vi "POST.vi"(6 "timeout":i32=10000, 7 "output file":path, 8 "error in":errorcluster, 9 "buffer":string, 10 "url":string, 11 "http-client in":refnum<class "http-client.lvclass">) -> (0 "error out":errorcluster, 1 "body":string, 2 "headers":string, 3 "http-client out":refnum<class "http-client.lvclass">)   [LabVIEW 2020, in "REST Client.lvlib" / "http-client.lvclass"]
uses:
  http-client.lvclass
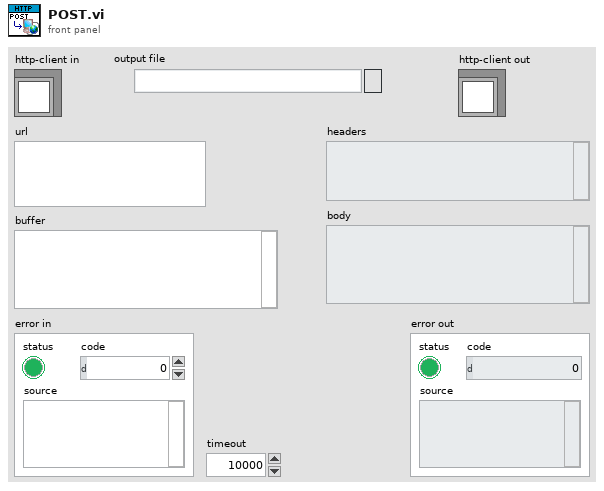
[diagram p1: front panel]
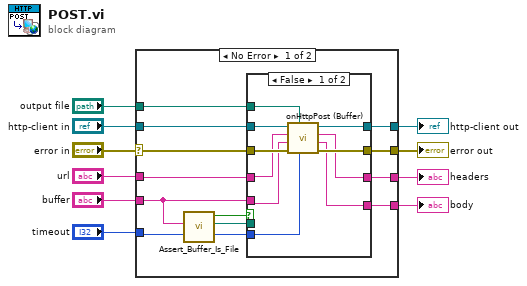
[diagram p0: block diagram]
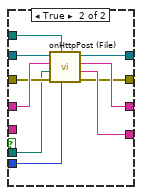
[diagram p2: hidden frame]
diagram:
  n1 = case shown="No Error" "error in" {
    selector: "error in" -> [w11 w44]
    tunnel: [w12 w44] -> w9
    tunnel: [w17 w43] -> w7
    tunnel: "http-client in" -> [w19 w43]
    tunnel: [w16 _] -> w6
    tunnel: "url" -> [w13 _]
    tunnel: "timeout" -> [w14 _]
    tunnel: "output file" -> [w18 _]
    tunnel: [w15 _] -> w2
    tunnel: "buffer" -> [w20 _]
    frame No Error {
      n2 = call "Assert_Buffer_Is_File.vi"("body"=w20) -> ("File"=w21:path, "is File?"=w22:bool)  [unwired: 9 in]
      n3 = case shown="False" w22 {
        tunnel: w21 -> [_ w33]
        tunnel: w20 -> [w28 _]
        tunnel: w19 -> [w32 w42]
        tunnel: w18 -> [w31 w41]
        tunnel: [w26 w40] -> w17
        tunnel: [w25 w39] -> w16
        tunnel: [w24 w38] -> w15
        tunnel: w14 -> [w23 w37]
        tunnel: w13 -> [w29 w36]
        tunnel: [w27 w35] -> w12
        tunnel: w11 -> [w30 w34]
        frame False {
          n4 = call-dynamic "onHttpPost (Buffer).vi"("timeout"=w23, "output file"=w31, "error in"=w30, "buffer"=w28, "url"=w29, "http-method in"=w32) -> ("error out"=w27:errorcluster, "body"=w24:string, "headers"=w25:string, "http-method out"=w26:refnum<class "http-client.lvclass">)  [unwired: 2 in]
        }
        frame True {
          n5 = call-dynamic "onHttpPost (File).vi"("timeout"=w37, "output file"=w41, "error in"=w34, "file"=w33, "url"=w36, "http-method in"=w42) -> ("error out"=w35:errorcluster, "body"=w38:string, "headers"=w39:string, "http-method out"=w40:refnum<class "http-client.lvclass">)  [unwired: 2 in]
        }
      }
    }
    frame Error {
    }
  }
  "error out" <- w9
  "http-client out" <- w7
  "headers" <- w6
  "body" <- w2
